vi "NEW.vi"() -> ()   [LabVIEW 2014]
uses:
  User Defined/I2C_Platform_Selector.ctl
  <vilib>/Instr/_visa.llb/VISA Open Access Mode.ctl
  <vilib>/MakerHub/LINX/Public/Peripherals/Digital/Digital Write 1 Chan.vi
  <vilib>/MakerHub/LINX/Public/Peripherals/Digital/Digital Write N Chans.vi
  <vilib>/MakerHub/LINX/Private/Local IO/LinxDigitalWrite.vi
  <vilib>/MakerHub/LINX/Public/Utilities/Check Channel.vi
  <vilib>/MakerHub/LINX/Private/Local IO/Handle Errors.vi
  <vilib>/MakerHub/LINX/Public/Utilities/Open Local.vi
  <vilib>/MakerHub/LINX/Private/Utilties/Generate Error.vi
  <vilib>/MakerHub/LINX/LMH-LINX.lvlib
  <vilib>/MakerHub/LINX/Public/Peripherals/UART/UART Write String.vi
  <vilib>/MakerHub/LINX/Public/Peripherals/UART/UART Read String.vi
panel:
  out "read buffer":string
  out "appended array":u8[](array[numeric]) format="%.0x"
  in  "I2C Slave Address (0) 2":u8=117 format="%.0x"
  in  "EXP2_Port1":bool[](array[boolean])
  in  "EXP2_Port0":bool[](array[boolean])
  in  "EXP1_Port 1":bool[](array[boolean])
  in  "EXP1_Port0":bool[](array[boolean])
  in  "GPIO4-":bool
  in  "GPIO22- UART":bool=TRUE
  out "Data":string
  in  "Flasher Programing":bool=TRUE
  in  "stop":bool
  in  "I2C Slave Address (0)":u8=116 format="%.0x"
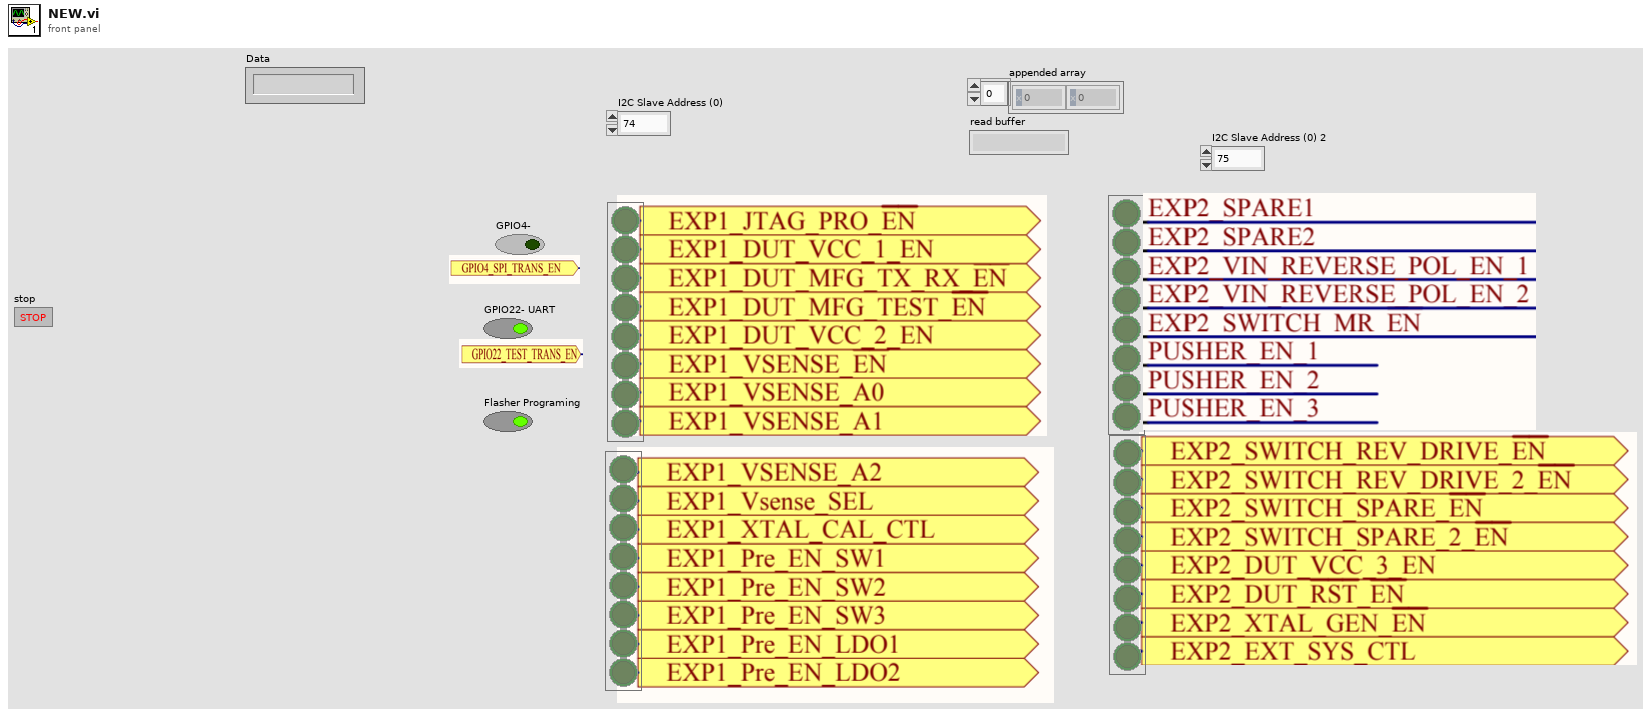
[diagram p1: front panel]
types:
  T1 = typedef "I2C_Platform_Selector.ctl" = enum16{"ESP8266-I2C", "Raspberry Pi-I2C"}
  T2 = typedef "LMH-LINX.lvlib/LINX Ref.ctl" = cluster{"IO":T3, "Interface":T4, "LINX Device Config":T5}
  T3 = typedef "LMH-LINX.lvlib/Platform.ctl" = enum16{"Remote", "Local"}
  T4 = typedef "LMH-LINX.lvlib/Interface.ctl" = enum16{"Serial", "TCP"}
  T5 = typedef "LMH-LINX.lvlib/Device.lvlib/LINX Device Config.ctl" = cluster{"Interface":T4, "COM Port":refnum<visa-resource-name>, "TCP Configuration":T6, "Device Family":u8, "Device ID":u8, "Device Name":string, "TCP Ref":refnum<k5>, "Channels":T7}
  T6 = typedef "LMH-LINX.lvlib/Device.lvlib/TCP Config.ctl" = cluster{"IP Address":string, "Port":u16}
  T7 = typedef "LMH-LINX.lvlib/Channels.ctl" = cluster{"DI":u8[], "DO":u8[], "AI":u8[], "AO":u8[], "PWM":u8[], "QE":u8[], "UART":u8[], "I2C 2":u8[], "SPI":u8[], "CAN":u8[], "Servo":u8[], "AI Ref (V)":dbl, "AI Resolution (Bits)":u8, "AO Ref (V)":dbl, "AO Resolution (Bits)":u8}
  T8 = typedef "VISA Open Access Mode.ctl" = u32
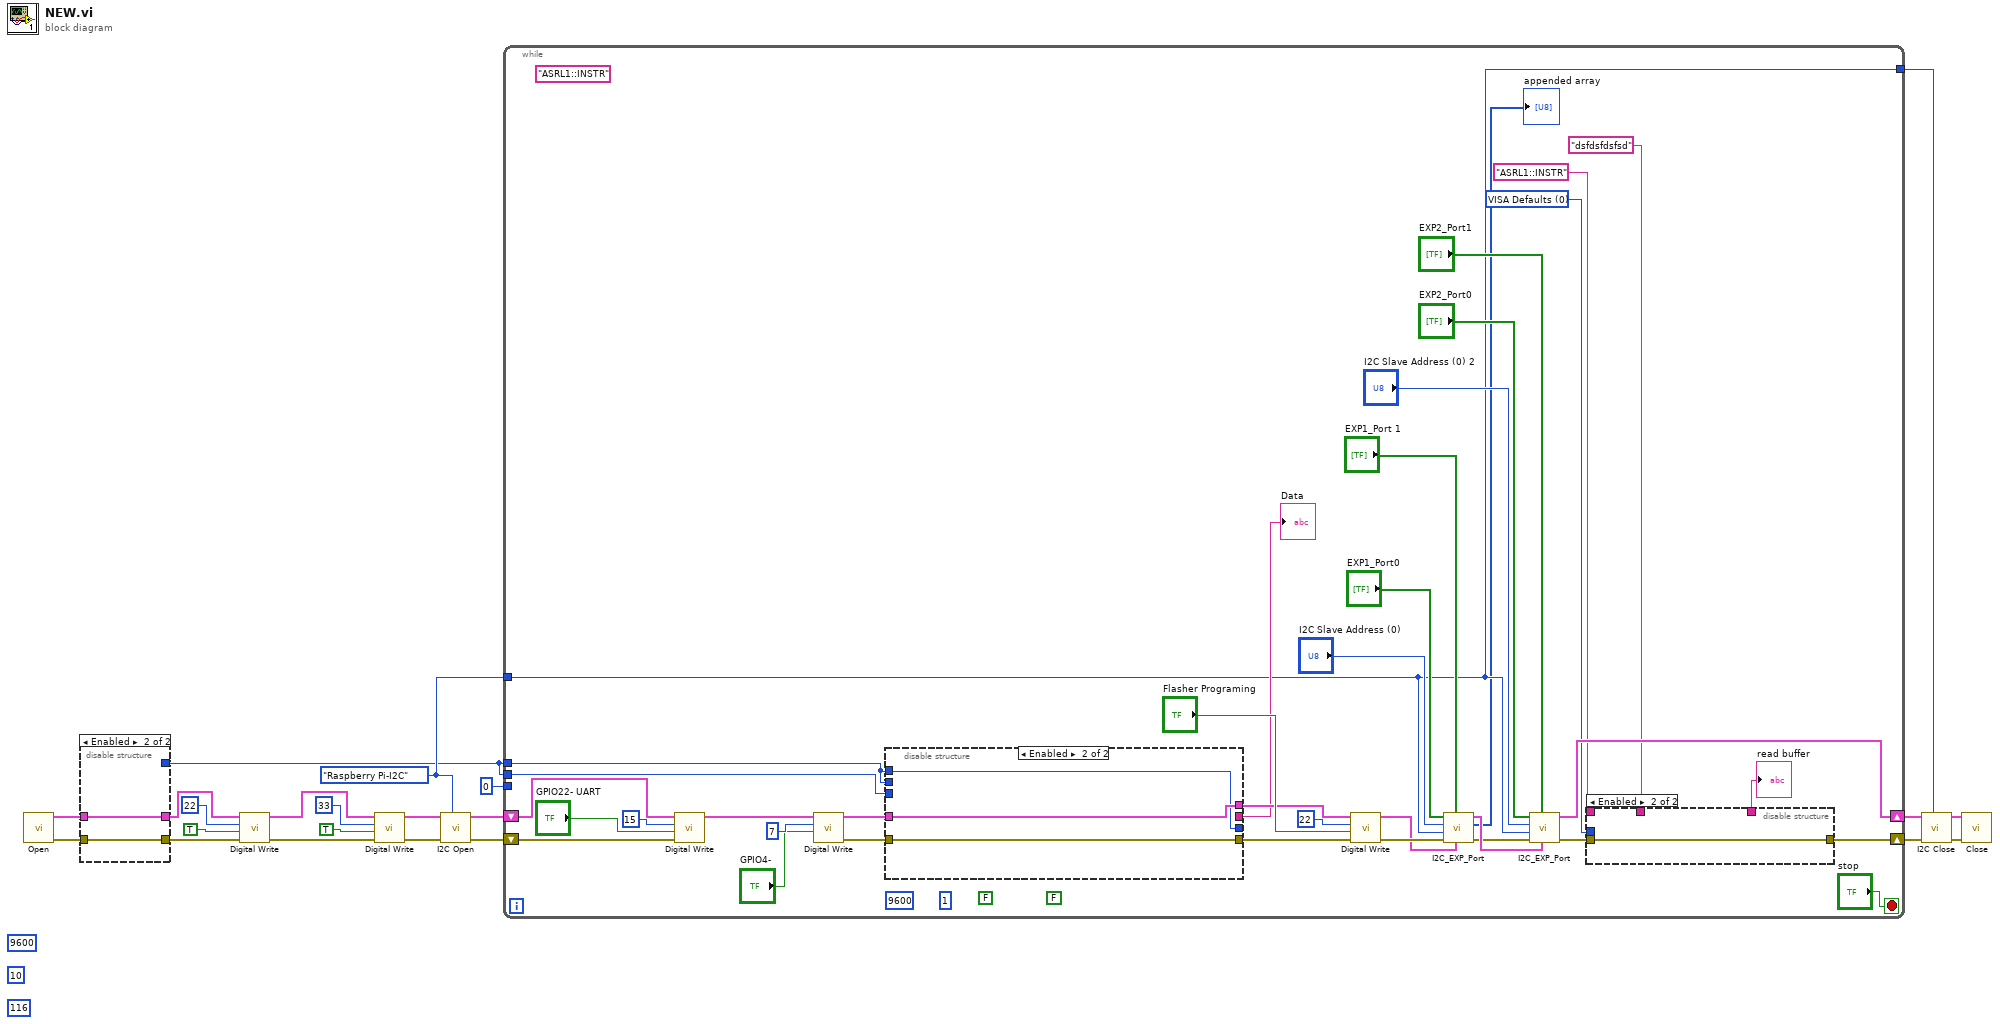
[diagram p0: block diagram]
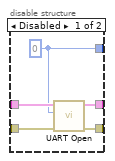
[diagram p2: hidden frame]
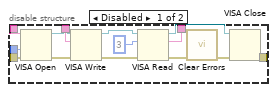
[diagram p3: hidden frame]
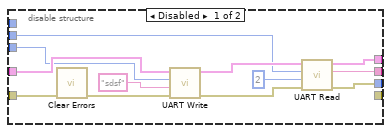
[diagram p4: hidden frame]
diagram:
  (unwired) u32 9600 ("Baud Rate (9600)")
  w9 = I2C_Platform_Selector."Raspberry Pi-I2C" ("I2C_Channel_platform")
  (unwired) 10
  (unwired) u8 116 ("I2C Slave Address (0)")
  n1 = call-poly <vilib>:"Open.vi"() -> ("Error Out"=w5:errorcluster, "LINX Resource"=w7:T2)  [unwired: 9 in, 1 out]
  n2 = disable-structure shown="Enabled" {
    disable-tunnel: w7 -> [w27 w29]
    disable-tunnel: [w26 w29] -> w6
    disable-tunnel: w5 -> [w25 w28]
    disable-tunnel: [w24 w28] -> w4
    disable-tunnel: [w23 _] -> w3
    frame Disabled {
      w23 = u8 0 ("UART Channel (0)")
      n3 = call <vilib>:"UART Open.vi"("Error In"=w25, "UART Channel (0)"=w23, "LINX Resource"=w27) -> ("Error Out"=w24:errorcluster, "LINX Resource"=w26:T2)  [unwired: 6 in, 1 out]
    }
    frame Enabled {
    }
  }
  n4 = call-poly <vilib>:"Digital Write.vi"("Error In"=w4, "Output Value"=TRUE ("Output Value 2"), "DO Channel"=u8 22 ("DO Channel 2"), "LINX Resource"=w6) -> ("Error Out"=w10:errorcluster, "LINX Resource"=w15:T2)  [unwired: 6 in]
  n5 = call-poly <vilib>:"Digital Write.vi"("Error In"=w10, "Output Value"=TRUE ("Output Value 2"), "DO Channel"=u8 33 ("DO Channel 2"), "LINX Resource"=w15) -> ("Error Out"=w11:errorcluster, "LINX Resource"=w14:T2)  [unwired: 6 in]
  n6 = call <vilib>:"I2C Open.vi"("I2C Channel (0)"=w9, "Error In"=w11, "LINX Resource"=w14) -> ("Error Out"=w12:errorcluster, "LINX Resource"=w13:T2)  [unwired: 7 in]
  n7 = while {
    tunnel: [w37] -> w18
    shift-right: [w30] -> w1
    shift-left: w12 -> [w51]
    shift-right: [w43] -> w2
    shift-left: w13 -> [w52]
    tunnel: w9 -> [w37]
    tunnel: u8 0 ("UART Channel (0)") -> [_]
    tunnel: w3 -> [w59]
    tunnel: w3 -> [w56]
    stop <- "stop" stop-if-true
    (unwired) "ASRL1::INSTR"
    w33 = T8 0 items=["VISA Defaults"=0, "Exclusive Lock"=1, "Load Configured Settings"=4] ("Access Mode")
    (unwired) u32 9600 ("Baud Rate Override")
    (unwired) u8 1 ("Num Bytes")
    (unwired) FALSE
    (unwired) FALSE
    n8 = call-poly <vilib>:"Digital Write.vi"("Error In"=w51, "Output Value"="GPIO22- UART", "DO Channel"=u8 15 ("DO Channel 2"), "LINX Resource"=w52) -> ("LINX Resource"=w47:T2)  [unwired: 6 in, 1 out]
    n9 = call-poly <vilib>:"Digital Write.vi"("Output Value"="GPIO4-", "DO Channel"=u8 7 ("DO Channel 2"), "LINX Resource"=w47) -> ("Error Out"=w48:errorcluster, "LINX Resource"=w49:T2)  [unwired: 7 in]
    n10 = disable-structure shown="Enabled" {
      disable-tunnel: w49 -> [w92 w95]
      disable-tunnel: w59 -> [w90 _]
      disable-tunnel: [w88 w95] -> w58
      disable-tunnel: [w87 _] -> w57
      disable-tunnel: [w86 w94] -> _
      disable-tunnel: w56 -> [w85 _]
      disable-tunnel: w48 -> [w82 w93]
      disable-tunnel: w56 -> [_ w94]
      disable-tunnel: [_ w93] -> w55
      frame Disabled {
        n11 = call <vilib>:"Clear Errors.vi"("error in (no error)"=w82) -> ("error out"=w81:errorcluster)  [unwired: 5 in, 1 out]
        n12 = call-poly <vilib>:"UART Write.vi"("Error In"=w81, "Data"="sdsf", "UART Channel (0)"=w90, "LINX Resource"=w92) -> ("Error Out"=w83:errorcluster, "LINX Resource"=w89:T2)  [unwired: 6 in]
        n13 = call-poly <vilib>:"UART Read.vi"("Error In"=w83, "Num Bytes"=u8 2, "UART Channel (0)"=w85, "LINX Resource"=w89) -> ("Error Out"=w86:errorcluster, "Data"=w87:string, "LINX Resource"=w88:T2)  [unwired: 5 in]
      }
      frame Enabled {
      }
    }
    "Data" <- w57
    n14 = call-poly <vilib>:"Digital Write.vi"("Error In"=w55, "Output Value"="Flasher Programing", "DO Channel"=u8 22 ("DO Channel 2"), "LINX Resource"=w58) -> ("Error Out"=w61:errorcluster, "LINX Resource"=w60:T2)  [unwired: 6 in]
    n15 = call "I2C_EXP_Port.vi"("LINX Resource in"=w60, "EXP1_Port 1"="EXP1_Port 1", "error in (no error)"=w61, "I2C_Channel_platform"=w37, "I2C Slave Address (0)"="I2C Slave Address (0)", "EXP1_Port0"="EXP1_Port0") -> ("error out"=w39:errorcluster, "appended array"=→"appended array":u8[], "LINX Resource out"=w40:T2)  [unwired: 3 in]
    n16 = call "I2C_EXP_Port.vi"("LINX Resource in"=w40, "EXP1_Port 1"="EXP2_Port1", "error in (no error)"=w39, "I2C_Channel_platform"=w37, "I2C Slave Address (0)"="I2C Slave Address (0) 2", "EXP1_Port0"="EXP2_Port0") -> ("error out"=w31:errorcluster, "LINX Resource out"=w43:T2)  [unwired: 3 in, 1 out]
    n17 = disable-structure shown="Enabled" {
      disable-tunnel: [w79 _] -> w35
      disable-tunnel: "dsfdsfdsfsd" ("write buffer") -> [w74 _]
      disable-tunnel: w33 -> [w71 _]
      disable-tunnel: "ASRL1::INSTR" -> [w70 _]
      disable-tunnel: w31 -> [w67 w80]
      disable-tunnel: [w66 w80] -> w30
      frame Disabled {
        n18 = VISA Open(access mode=w71, error in (no error)=w67, VISA resource name=w70) -> (VISA resource name=w72:refnum<visa-resource-name>, error out=w73:errorcluster)  [unwired: 2 in]
        n19 = VISA Write(VISA resource name=w72, write buffer=w74, error in (no error)=w73) -> (VISA resource name out=w75:refnum<visa-resource-name>, error out=w76:errorcluster)  [unwired: 1 out]
        n20 = VISA Read(VISA resource name=w75, byte count=u32 3, error in (no error)=w76) -> (VISA resource name out=w77:refnum<visa-resource-name>, read buffer=w79:string, error out=w69:errorcluster)  [unwired: 1 out]
        n21 = call <vilib>:"Clear Errors.vi"("error in (no error)"=w69) -> ("error out"=w68:errorcluster)  [unwired: 5 in, 1 out]
        n22 = VISA Close(VISA resource name=w77, error in (no error)=w68) -> (error out=w66:errorcluster)
      }
      frame Enabled {
      }
    }
    "read buffer" <- w35
  }
  n23 = call <vilib>:"I2C Close.vi"("I2C Channel (0)"=w18, "Error In"=w1, "LINX Resource"=w2) -> ("Error Out"=w21:errorcluster, "LINX Resource"=w22:T2)  [unwired: 7 in]
  n24 = call <vilib>:"Close.vi"("Error In"=w21, "LINX Resource"=w22) -> ()  [unwired: 9 in, 1 out]
